vi "Translate.vi"(0 "Angle (Rad)":dbl, 1 "Execute":bool=TRUE, 2 "Distance (Feet)":dbl=10.0, 3 "Percent Speed":dbl=0.8) -> (4 "Done Executing":bool)   [LabVIEW 2011]
uses:
  Globals/Max Robot Speed.vi
  Globals/Encoders Global.vi
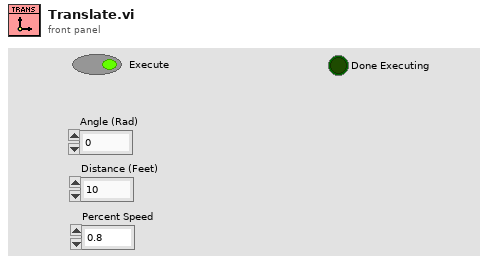
[diagram p1: front panel]
types:
  T1 = typedef "WPI_EncoderDevRef.ctl" = cluster{"DevStatus":errorcluster, "EncoderIndex":T2, "CounterIndex":T3, "DistancePerCount":dbl, "Decoding Type":T4}
  T2 = typedef "FPGA_EncoderIdx.ctl" = enum8{"Enc 0", "Enc 1", "Enc 2", "Enc 3", "Invalid"}
  T3 = typedef "FPGA_CounterCtrSystemIndex.ctl" = enum8{"Ctr 0", "Ctr 1", "Ctr 2", "Ctr 3", "Ctr 4", "Ctr 5", "Ctr 6", "Ctr 7", "Invalid"}
  T4 = typedef "WPI_EncoderType.ctl" = enum16{"1x", "2x", "4x"}
  T5 = cluster{"Front Left":T1, "Front Right":T1, "Rear Left":T1, "Rear Right":T1, "Shooter":T1}
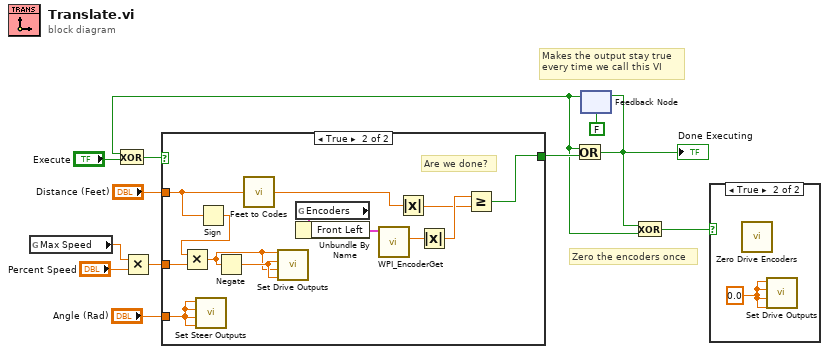
[diagram p0: block diagram]
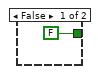
[diagram p3: hidden frame]
diagram:
  # "Makes the output stay true\nevery time we call this VI"
  # "Zero the encoders once"
  n1 = global read "Max Robot Speed.vi" "Max Speed"() -> (w2:dbl)
  n2 = Multiply(x=w2, y="Percent Speed") -> (x*y=w3:dbl)
  n3 = feedback #1(FALSE) -> (w5:bool)
  n4 = Exclusive Or(1:"Execute", 2:w5) -> (0:w12:bool)
  n5 = case shown="True" w12 {
    tunnel: [FALSE w26] -> w10
    tunnel: "Angle (Rad)" -> [_ w24]
    tunnel: w3 -> [_ w19]
    tunnel: "Distance (Feet)" -> [_ w18]
    frame False {
    }
    frame True {
      # "Are we done?"
      n6 = call "Set Steer Outputs.vi"("Rear Right"=w24, "Rear Left"=w24, "Front Right"=w24, "Front Left"=w24) -> ()  [unwired: 8 in]
      n7 = Sign(1:w18) -> (0:w16:dbl)
      n8 = Multiply(x=w16, y=w19) -> (x*y=w17:dbl)
      n9 = Negate(x=w17) -> (-x=w20:dbl)
      n10 = call "Feet to Codes.vi"("Feet"=w18) -> ("Codes"=w25:dbl)
      n11 = call "Set Drive Outputs.vi"("Rear Right"=w20, "Rear Left"=w17, "Front Right"=w20, "Front Left"=w17) -> ()  [unwired: 8 in]
      n12 = global read "Encoders Global.vi" "Encoders"() -> (w23:T5)
      n13 = Unbundle By Name(w23) -> ("Front Left"=w22:T1)
      n14 = call <vilib>:"WPI_EncoderGet.vi"("EncoderDevRef"=w22) -> ("Distance"=w21:dbl)  [unwired: 5 in, 5 out]
      n15 = Absolute Value(x=w25) -> (abs(x)=w14:dbl)
      n16 = Absolute Value(x=w21) -> (abs(x)=w15:dbl)
      n17 = Greater Or Equal?(x=w15, y=w14) -> (x >= y?=w26:bool)
    }
  }
  n18 = Or(x=w5, y=w10) -> (x .or. y?=w4:bool)
  "Done Executing" <- w4
  n19 = feedback-in #1(w4) -> ()
  n20 = Exclusive Or(1:w5, 2:w4) -> (0:w6:bool)
  n21 = case shown="True" w6 {
    frame False {
    }
    frame True {
      w27 = 0.0
      n22 = call "Zero Drive Encoders.vi"() -> ()  [unwired: 12 in]
      n23 = call "Set Drive Outputs.vi"("Rear Right"=w27, "Rear Left"=w27, "Front Right"=w27, "Front Left"=w27) -> ()  [unwired: 8 in]
    }
  }
